vi "Push to Stack.vi"(8 "error in (no error)":errorcluster caption="错误输入（无错误）", 10 "Element":variant, 11 "Stack 输入":refnum<class "Stack.lvclass"> caption="DNL_LabVIEW Object in") -> (0 "error out":errorcluster caption="错误输出", 3 "Stack 输出":refnum<class "Stack.lvclass"> caption="DNL_LabVIEW Object out")   [LabVIEW 2011, in "Stack.lvclass"]
uses:
  Stack.lvclass
  Stack.lvclass/Stack.ctl
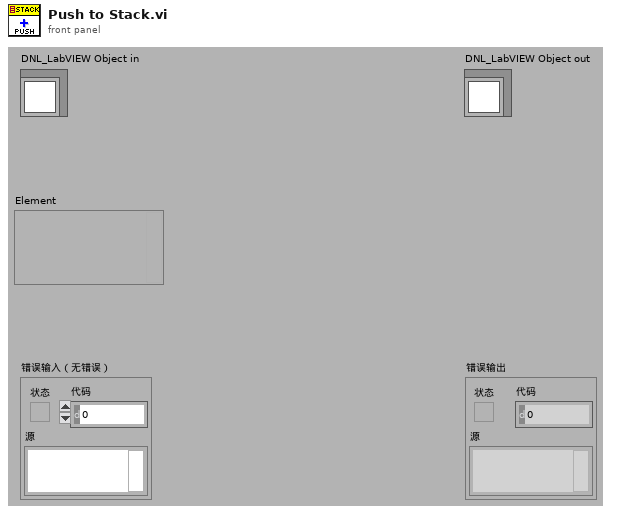
[diagram p1: front panel]
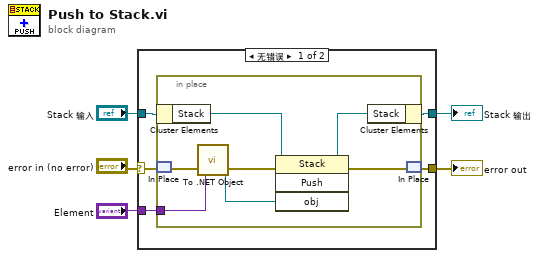
[diagram p0: block diagram]
diagram:
  n1 = case shown="无错误" "error in (no error)" {
    selector: "error in (no error)" -> [w7 w19]
    tunnel: [w6 w19] -> w4
    tunnel: [w8 w18] -> w2
    tunnel: "Stack 输入" -> [w10 w18]
    tunnel: "Element" -> [w9 _]
    frame No Error {
      n2 = in-place {
        in-place-border: w9 -> [w14]
        n3 = in-place-cluster #1(w10) -> ("Stack"=w17:refnum<k24>)
        n4 = in-place-match #2(w7) -> (w13:errorcluster)
        n5 = call <vilib>:"To .NET Object.vi"("error in (no error)"=w13, "anything"=w14) -> ("error out"=w12:errorcluster, ".NET object"=w15:refnum<k24>)
        n6 = invoke class="Stack" method="Push"(reference=w17, error in=w12, "obj"=w15) -> (reference out=w16:refnum<k24>, error out=w11:errorcluster)  [unwired: 1 in, 2 out]
        n7 = in-place-cluster #1("Stack"=w16) -> (w8:refnum<class "Stack.lvclass">)
        n8 = in-place-match #2(w11) -> (w6:errorcluster)
      }
    }
    frame Error {
    }
  }
  "error out" <- w4
  "Stack 输出" <- w2
